vi "IsString.vi"(4 "Value String in":string) -> (0 "IsString":bool, 2 "String Value":string)   [LabVIEW 2019]
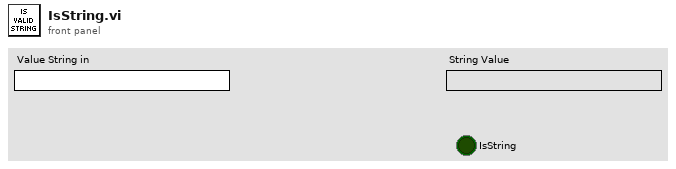
[diagram p1: front panel]
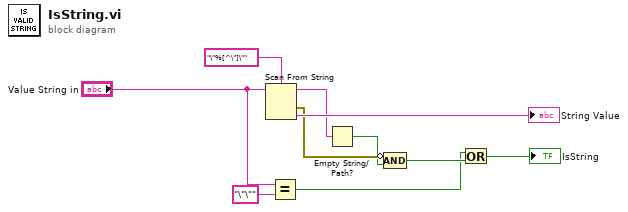
[diagram p0: block diagram]
diagram:
  n1 = Scan From String(format string="\"%[^\"]\"", input string="Value String in") -> (remaining string=w6:string, error out=w7:errorcluster, output 1=→"String Value":string)  [unwired: 3 in, 1 out]
  n2 = Equal?(x="Value String in", y="\"\"") -> (x = y?=w1:bool)
  n3 = Empty String/Path?(string/path=w6) -> (empty?=w5:bool)
  n4 = Compound Arithmetic op=AND(invert w7, w5) -> (w9:bool)
  n5 = Or(x=w1, y=w9) -> (x .or. y?=→"IsString":bool)
